vi "FTW-CodeGen-FindTerm-Adaptive.vi"(5 "AdaptiveTerms":T1[](array[typedef]), 7 "Terminal ID":string) -> (4 "Index":i32, 6 "AdaptiveTerm":T1={"Config"={"AllowedTypes"=[], "UnconstrainedTypeBehavior"=enum."UseDefaultType", "DefaultType"=variant}, "ID"="", "ParentIndex"=0, "Wired?"=FALSE, "WiredTypeAllowed?"=FALSE, "LastValidWireName"="", "LastValidWireType"=enum."Array", "Followers"=[]}, 8 "Found?":bool)   [LabVIEW 2015]
uses:
  FTW-CodeGen-XNodeAdaptiveTerminal.ctl
  FTW-CodeGen-XNodeAdaptiveTerminal-Controller.ctl
  src/reflection/FTW-Reflection-Types.ctl
  FTW-CodeGen-XNodeAdaptiveTerminal-ControllerBehavior.ctl
panel:
  # "Inputs"
  # "Outputs"
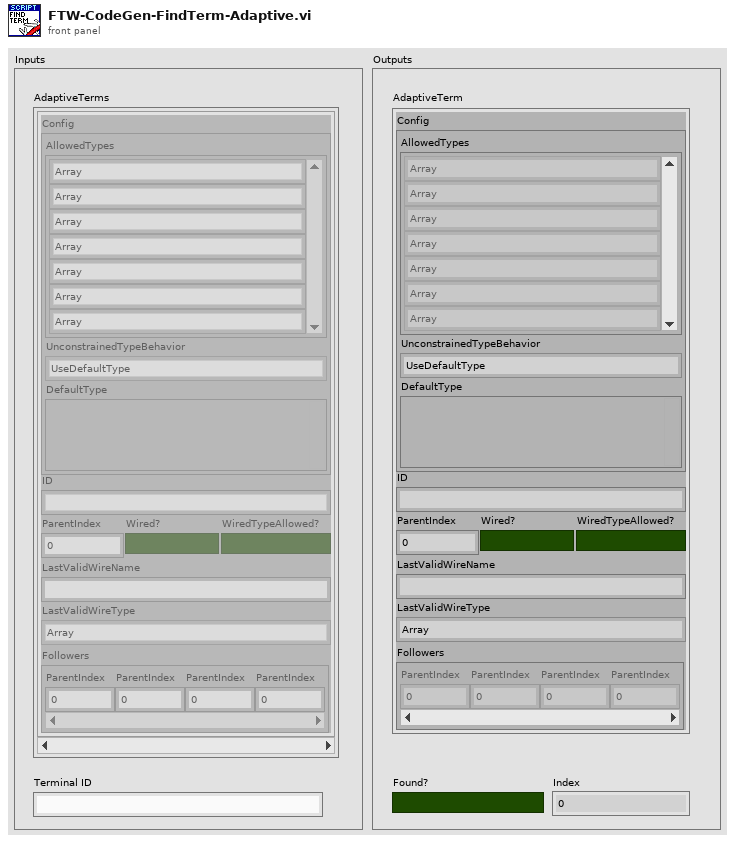
[diagram p1: front panel]
types:
  T1 = typedef "FTW-CodeGen-XNodeAdaptiveTerminal.ctl" = cluster{"Config":T2, "ID":string, "ParentIndex":i32, "Wired?":bool, "WiredTypeAllowed?":bool, "LastValidWireName":string, "LastValidWireType":T3, "Followers":i32[]}
  T2 = typedef "FTW-CodeGen-XNodeAdaptiveTerminal-Controller.ctl" = cluster{"AllowedTypes":T3[], "UnconstrainedTypeBehavior":T4, "DefaultType":variant}
  T3 = typedef "FTW-Reflection-Types.ctl" = enum16{"Unknown", "Void", "Array", "Cluster", "LVObject", "Boolean", "I8", "I16", "I32", "I64", "U8", "U16", "U32", "U64", "SGL", "DBL", "EXT", "CSG", "CDB", "CXT", "FXP", "EnumU8", "EnumU16", "EnumU32", "EnumU64", "SGLwithUnit", "DBLwithUnit", "EXTwithUnit", "CSGwithUnit", "CDBwithUnit", "CXTwithUnit", "String", "Path", "Picture", "Tag", "LVVariant", "Timestamp", "WaveformI8", "WaveformI16", "WaveformI32", "WaveformI64", "WaveformU8", "WaveformU16", "WaveformU32", "WaveformU64", "WaveformSGL", "WaveformDBL", "WaveformEXT", "WaveformCSG", "WaveformCDB", "WaveformCXT", "WaveformDigital", "WaveformUnknownType", "DigitalData", "DynamicData", "ExternalData", "FileByteStream", "TDMStream", "dotNET", "ActiveX", "VIServerReference", "VIReference", "ApplicationInstance", "Menu", "ConnectionDataSocket", "ConnectionVISA", "ConnectionBluetooth", "ConnectionIrDA", "ConnectionTCP", "ConnectionUDP", "ConnectionHTTPClient", "ConnectionFTP", "Occurrence", "Notifier", "Queue", "Rendezvous", "Semaphore", "RTFIFO", "EventPublisher", "EventRegistration", "EventCallback", "DataValueReference", "GenericClass", "GenericClassTag", "GenericClassDeepCopy", "GenericClassFlattened", "GenericClassTagFlattened", "GenericReferenceType", "WindowsRegistry", "OverloadedDatalogRef", "ReferenceUnknownType", "ByteArray", "ConPaneInterface", "FTWObject"}
  T4 = typedef "FTW-CodeGen-XNodeAdaptiveTerminal-ControllerBehavior.ctl" = enum16{"UseDefaultType", "StickyToLastValidType"}
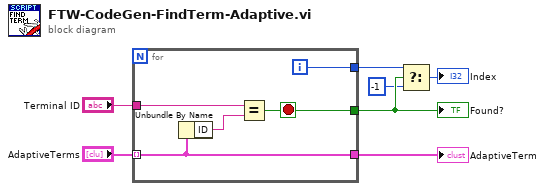
[diagram p0: block diagram]
diagram:
  n1 = for {
    tunnel: [w9] -> w6
    tunnel: [w12] -> w4
    tunnel: "AdaptiveTerms" -> [w9] mode=indexing
    tunnel: "Terminal ID" -> [w10]
    tunnel: [w8] -> w3
    i -> [w8]
    stop <- w12 stop-if-true
    n2 = Unbundle By Name(w9) -> ("ID"=w11:string)
    n3 = Equal?(x=w10, y=w11) -> (x = y?=w12:bool)
  }
  "AdaptiveTerm" <- w6
  "Found?" <- w4
  n4 = Select(t=w3, s=w4, f=-1) -> (s? t:f=→"Index":i32)
